vi "sub_decision_main.vi"(8 "error in":errorcluster) -> (0 "error out":errorcluster)   [LabVIEW 2019]
uses:
  _ctrl/create-rw-close.ctl
  _ctrl/rw.ctl
  <vilib>/measure/mascope.llb/Transition Measurements N chan.vi
  <vilib>/measure/NI_MAPro.lvlib
panel:
  out "DL950":waveform(dbl)[](graph)
  out "숫자형":i32
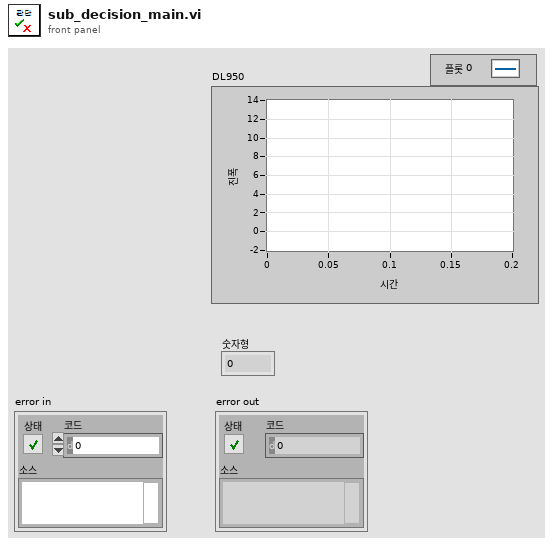
[diagram p1: front panel]
types:
  T1 = typedef "create-rw-close.ctl" = enum16{"create", "write", "read", "delete", "close"}
  T2 = typedef "rw.ctl" = enum16{"read", "write"}
  T3 = typedef "DL950_wfms.ctl" = cluster{"wfms":waveform(dbl)[], "Waveform_2":cluster{"t0":dbl, "dt":dbl, "Y":dbl[][]}, "items":dbl[][], "da950_array":dbl[]}
  T4 = typedef "ref_all.ctl" = cluster{"DL950_config":refnum<vi>, "BP4610 Config":refnum<vi>, "DSP1950 Config":refnum<vi>, "2470-config":refnum<vi>, "cDAQ 9269 AO config":refnum<vi>, "cDAQ 9221 Config":refnum<vi>, "cDAQ-9467 Config":refnum<vi>, "Waveform":refnum<vi>, "DL950 wfm":refnum<vi>, "AI Graph":refnum<vi>, "AO_Wave-config":refnum<vi>, "DL950 items":refnum<vi>, "Volt":refnum<vi>, "Current":refnum<vi>, "AO_Level":refnum<vi>, "RC-Testconfig":refnum<vi>, "RC-Test Judgement ":refnum<vi>, "Log path":refnum<vi>, "시험명":refnum<vi>, "file renew[Hr]":refnum<vi>, "Breakdown-Spec":refnum<vi>}
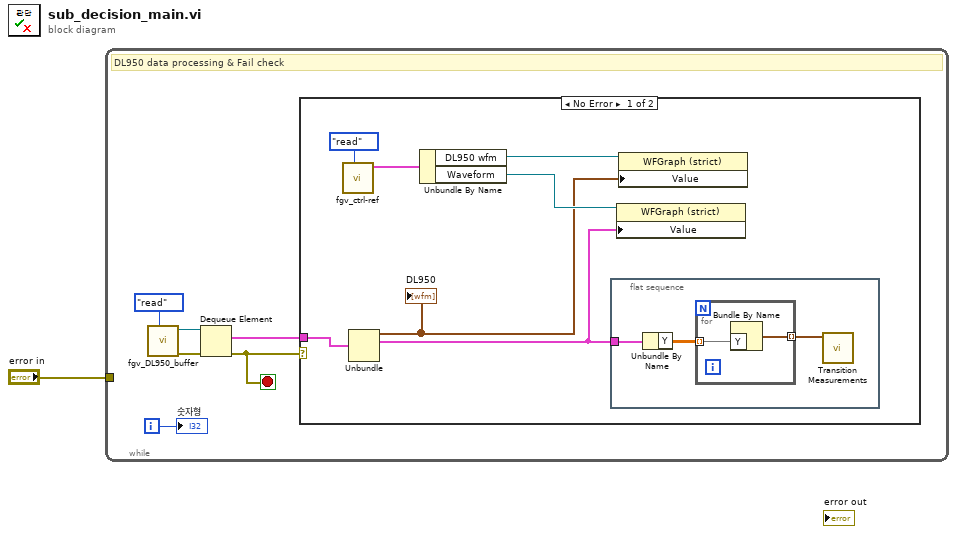
[diagram p0: block diagram]
diagram:
  n1 = while {
    tunnel: "error in" -> [_]
    i -> [w2]
    stop <- w4 stop-if-true
    # "DL950 data processing & Fail check"
    n2 = call "fgv_DL950_buffer.vi"("cmd"=create-rw-close."read") -> ("error out"=w6:errorcluster, "queue out"=w5:refnum<queue>)  [unwired: 9 in]
    n3 = Dequeue Element(queue=w5, error in (no error)=w6) -> (element=w3:T3, error out=w4:errorcluster)  [unwired: 1 in, 2 out]
    n4 = case shown="No Error" w4 {
      tunnel: w3 -> [w10 _]
      frame No Error {
        n5 = call "fgv_ctrl-ref.vi"("cmd"=rw."read") -> ("output cluster 2"=w13:T4)  [unwired: 9 in, 1 out]
        n6 = Unbundle(w10) -> ("wfms"=w9:waveform(dbl)[], "Waveform_2"=w8:cluster{"t0":dbl, "dt":dbl, "Y":dbl[][]})  [unwired: 2 out]
        "DL950" <- w9
        n7 = Unbundle By Name(w13) -> ("DL950 wfm"=w12:refnum<vi>, "Waveform"=w11:refnum<vi>)
        n8 = flat-sequence {
          tunnel: w8 -> [w17]
          frame #0 {
            n9 = Unbundle By Name(w17) -> ("Y"=w16:dbl[][])
            n10 = for {
              tunnel: w16 -> [w19] mode=indexing
              tunnel: [w18] -> w15 mode=indexing
              n11 = Bundle By Name("Y"=w19) -> (w18:waveform(dbl))  [unwired: 1 in]
            }
            n12 = call-poly <vilib>:"Transition Measurements.vi"("signal(s) in"=w15) -> ()  [unwired: 5 in, 6 out]
          }
        }
        n13 = property class="WFGraph (strict)"(reference=w11, "Value"=w8) -> ()  [unwired: 1 in, 2 out]
        n14 = property class="WFGraph (strict)"(reference=w12, "Value"=w9) -> ()  [unwired: 1 in, 2 out]
      }
      frame Error {
      }
    }
    "숫자형" <- w2
  }
